vi "Convert Callback To Selected Item.vi"(6 "Return Meet Filter Selection (T)":bool=TRUE, 8 "error in":errorcluster, 10 "Data":variant, 11 "TreeAliasBrowser Ref":T1) -> (0 "error out":errorcluster, 3 "Selected Items":T2[](array[typedef]))   [LabVIEW 2020, in "NI_VS UI Tree Alias Browser.lvlib"]
uses:
  <vilib>/NI VeriStand/UI Controls/Tree and Alias Browser/NI_VS UI Tree Alias Browser.lvlib
  <vilib>/NI VeriStand/UI Controls/Tree and Alias Browser/Node Ref.ctl
  NationalInstruments.VeriStand.SystemStorage
  <vilib>/NI VeriStand/UI Controls/Tree and Alias Browser/Tree Alias Browser Ref.ctl
  NationalInstruments.VeriStand.SystemStorageUI
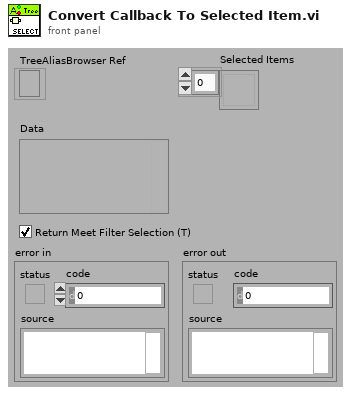
[diagram p1: front panel]
types:
  T1 = typedef "NI_VS UI Tree Alias Browser.lvlib/Tree Alias Browser Ref.ctl" = refnum<k24>
  T2 = typedef "NI_VS UI Tree Alias Browser.lvlib/Node Ref.ctl" = refnum<k24>
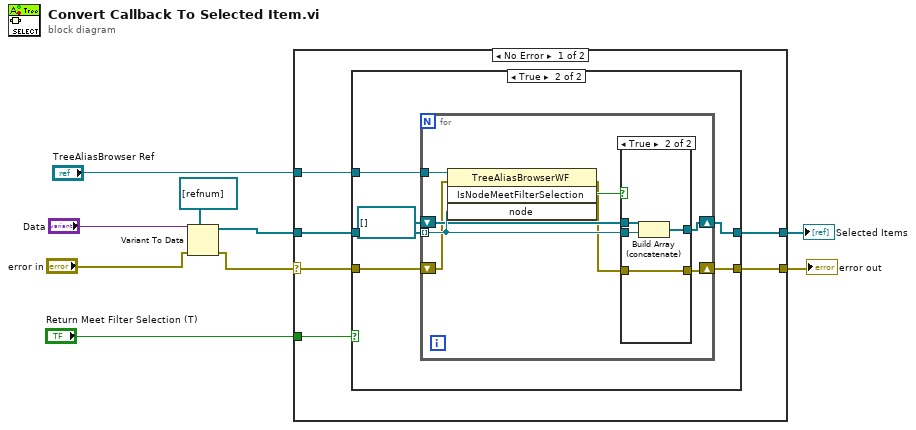
[diagram p0: block diagram]
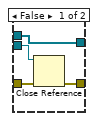
[diagram p3: hidden frame]
diagram:
  n1 = Variant To Data(error in="error in", type=T2[] [refnum] ("Selected Item"), Variant="Data") -> (data=w4:T2[], error out=w6:errorcluster)
  n2 = case shown="No Error" w6 {
    selector: w6 -> [w11 w41]
    tunnel: "TreeAliasBrowser Ref" -> [w15 _]
    tunnel: w4 -> [w13 w40]
    tunnel: "Return Meet Filter Selection (T)" -> [w14 _]
    tunnel: [w12 w40] -> w2
    tunnel: [w10 w41] -> w1
    frame No Error {
      n3 = case shown="True" w14 {
        tunnel: w15 -> [_ w23]
        tunnel: w13 -> [w17 w22]
        tunnel: [w17 w21] -> w12
        tunnel: w11 -> [w16 w19]
        tunnel: [w16 w18] -> w10
        frame False {
        }
        frame True {
          n4 = for {
            tunnel: w23 -> [w31]
            tunnel: w22 -> [w29] mode=indexing
            shift-right: [w28] -> w21
            shift-left: T2[] [] -> [w27]
            shift-right: [w24] -> w18
            shift-left: w19 -> [w26]
            n5 = invoke class="TreeAliasBrowserWF" method="IsNodeMeetFilterSelection"(reference=w31, error in=w26, "node"=w29) -> (error out=w25:errorcluster, "IsNodeMeetFilterSelection"=w30:bool)  [unwired: 1 in, 2 out]
            n6 = case shown="True" w30 {
              tunnel: w29 -> [w34 w39]
              tunnel: [w35 w38] -> w28
              tunnel: w27 -> [w35 w37]
              tunnel: w25 -> [w33 w36]
              tunnel: [w32 w36] -> w24
              frame False {
                n7 = Close Reference(reference=w34, error in (no error)=w33) -> (error out=w32:errorcluster)
              }
              frame True {
                n8 = Build Array (concatenate)(w37, w39) -> (w38:T2[])
              }
            }
          }
        }
      }
    }
    frame Error {
    }
  }
  "error out" <- w1
  "Selected Items" <- w2
